vi "Write Skip.vi"(8 "error in (no error)":errorcluster, 10 "Skip":bool, 11 "StepNode in":refnum<class "StepNode.lvclass">) -> (0 "error out":errorcluster, 3 "StepNode out":refnum<class "StepNode.lvclass">)   [LabVIEW 2015, in "StepNode.lvclass"]
uses:
  StepNode.lvclass
  Prototype/classes/Step/Config/Step Config.lvclass
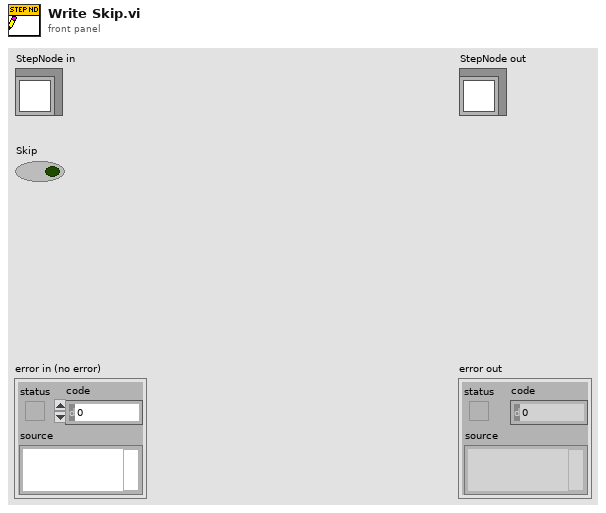
[diagram p1: front panel]
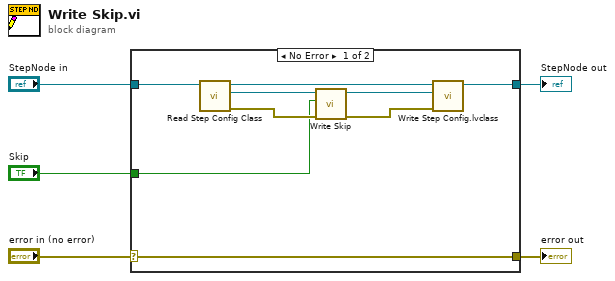
[diagram p0: block diagram]
diagram:
  n1 = case shown="No Error" "error in (no error)" {
    selector: "error in (no error)" -> [w14 w15]
    tunnel: [w14 w15] -> w4
    tunnel: [w12 w16] -> w2
    tunnel: "StepNode in" -> [w13 w16]
    tunnel: "Skip" -> [w6 _]
    frame No Error {
      n2 = call-dynamic "Read Step Config Class.vi"("StepNode in"=w13) -> ("error out"=w10:errorcluster, "Step Config.lvclass"=w8:refnum<class "Step Config.lvclass">, "StepNode out"=w11:refnum<class "StepNode.lvclass">)  [unwired: 8 in]
      n3 = call-dynamic "Write Skip.vi"("error in (no error)"=w10, "Skip"=w6, "Step Config in"=w8) -> ("error out"=w9:errorcluster, "Step Config out"=w7:refnum<class "Step Config.lvclass">)  [unwired: 7 in]
      n4 = call-dynamic "Write Step Config.lvclass.vi"("error in (no error)"=w9, "Step Config.lvclass"=w7, "StepNode in"=w11) -> ("StepNode out"=w12:refnum<class "StepNode.lvclass">)  [unwired: 7 in, 1 out]
    }
    frame Error {
    }
  }
  "error out" <- w4
  "StepNode out" <- w2
